vi "Diag Convertor.vi"(11 "diagonal":T2 items=["Non-unit", "Unit"]) -> (3 "diag":T1=131 items=["CblasNonUnit"=131, "CblasUnit"=132])   [LabVIEW 2020, in "NI_AALBLAS.lvlib"]
uses:
  <vilib>/Analysis/NI_AALBLAS.lvlib
  <vilib>/Analysis/BLAS.llb/LV_Diag.ctl
  <vilib>/Analysis/BLAS.llb/Diag.ctl
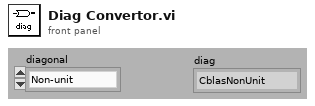
[diagram p1: front panel]
types:
  T1 = typedef "NI_AALBLAS.lvlib/Diag.ctl" = i32
  T2 = typedef "NI_AALBLAS.lvlib/LV_Diag.ctl" = i32
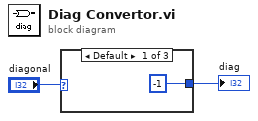
[diagram p0: block diagram]
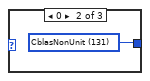
[diagram p2: hidden frame]
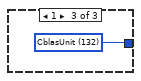
[diagram p3: hidden frame]
diagram:
  n1 = case shown="Default" "diagonal" {
    tunnel: [-1 w4 w5] -> w2
    frame Default {
    }
    frame 0 {
      w4 = T1 131 items=["CblasNonUnit"=131, "CblasUnit"=132] ("diag 2")
    }
    frame 1 {
      w5 = T1 132 items=["CblasNonUnit"=131, "CblasUnit"=132] ("diag 2")
    }
  }
  "diag" <- w2
